vi "getSignalRateLimit.vi"(8 "error in":errorcluster, 10 "Slave Address (7-bit)":u8, 11 "I2C Ref In":T1) -> (0 "error out":errorcluster, 2 "Mcps":dbl, 3 "I2C Ref Out":T1)   [LabVIEW 2018]
uses:
  <vilib>/myRIO/Instrument Drivers/Onboard IO/I2C/typedefs/I2C Reference.ctl
  <vilib>/myRIO/Common/Instrument Driver Framework/Utilities/typedefs/myRIO Generic Hardware Reference.ctl
  <vilib>/myRIO/Common/Instrument Driver Framework/Utilities/typedefs/Hardware Version Enum.ctl
  <vilib>/myRIO/Common/Instrument Driver Framework/Utilities/typedefs/myRIO v1.0 Reference.ctl
  <vilib>/myRIO/Common/Instrument Driver Framework/Utilities/typedefs/Generic FPGA Reference.ctl
  <vilib>/myRIO/Common/Instrument Driver Framework/myRIO v1.0/I2C/typedefs/I2C Channels Enum.ctl
  <vilib>/myRIO/Instrument Drivers/Onboard IO/I2C/typedefs/I2C Configuration.ctl
  <vilib>/myRIO/Instrument Drivers/Onboard IO/I2C/typedefs/I2C Transfer Rate.ctl
  <vilib>/Utility/error.llb/Error Cluster From Error Code.vi
  <vilib>/myRIO/Common/Instrument Driver Framework/myRIO v1.0/I2C/vis/myRIO v1.0 Write I2C.vi
  <vilib>/myRIO/Common/Instrument Driver Framework/myRIO v1.0/I2C/vis/myRIO v1.0 Read I2C.vi
  <vilib>/myRIO/Instrument Drivers/Onboard IO/I2C/I2C.lvlib
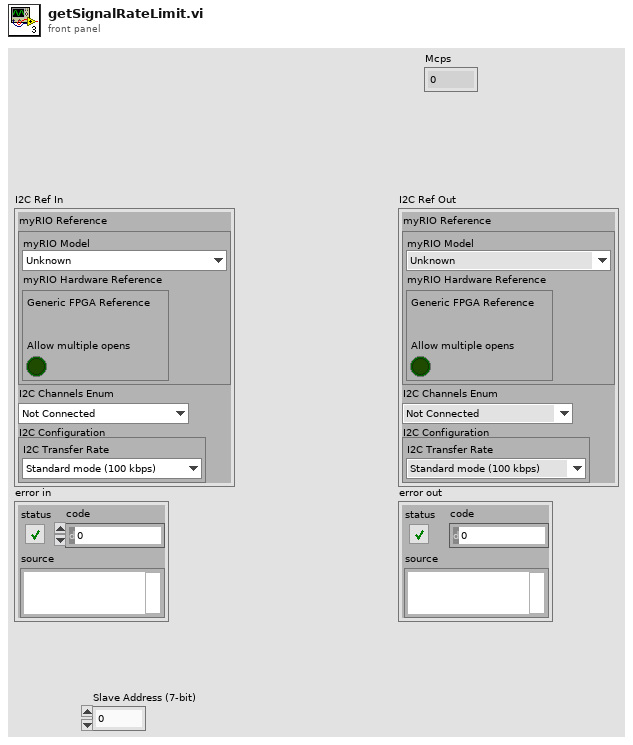
[diagram p1: front panel]
types:
  T1 = typedef "I2C.lvlib/I2C Reference.ctl" = cluster{"myRIO Reference":T2, "I2C Channels Enum":T6, "I2C Configuration":T7}
  T2 = typedef "myRIO Generic Hardware Reference.ctl" = cluster{"myRIO Model":T3, "myRIO Hardware Reference":T4}
  T3 = typedef "Hardware Version Enum.ctl" = enum16{"Unknown", "myRIO-1900", "myRIO-1950", "roboRIO", "NI ELVIS RIO CM", "ELVIS III"}
  T4 = typedef "myRIO v1.0 Reference.ctl" = cluster{"Generic FPGA Reference":T5, "Allow multiple opens":bool}
  T5 = typedef "Generic FPGA Reference.ctl" = refnum<k20>
  T6 = typedef "I2C Channels Enum.ctl" = enum16{"Not Connected", "A/I2C", "B/I2C", "I2C/I2C"}
  T7 = typedef "I2C.lvlib/I2C Configuration.ctl" = cluster{"I2C Transfer Rate":T8}
  T8 = typedef "I2C.lvlib/I2C Transfer Rate.ctl" = enum16{"Standard mode (100 kbps)", "Fast mode (400 kbps)"}
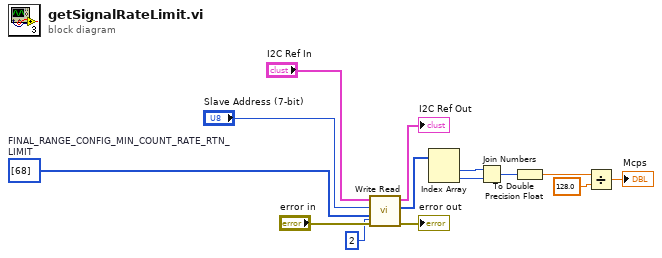
[diagram p0: block diagram]
diagram:
  w9 = u8[] [68]  # FINAL_RANGE_CONFIG_MIN_COUNT_RATE_RTN_LIMIT
  n1 = call <vilib>:"Write Read.vi"("Byte Count"=u32 2, "error in (no error)"="error in", "Bytes to Write"=w9, "Slave Address (7-bit)"="Slave Address (7-bit)", "I2C Ref In"="I2C Ref In") -> ("error out"=→"error out":errorcluster, "Bytes Read"=w7:u8[], "I2C Ref Out"=→"I2C Ref Out":T1)  [unwired: 3 in]
  n2 = Index Array(array=w7) -> (element #1=w6:u8, element #2=w5:u8)  [unwired: 2 in]
  n3 = Join Numbers(hi=w6, lo=w5) -> ((hi.lo)=w4:u16)
  n4 = To Double Precision Float(number=w4) -> (double precision float=w3:dbl)
  n5 = Divide(x=w3, y=128.0) -> (x/y=→"Mcps":dbl)
